vi "Balance.vi"(8 "Start Time":dbl, 10 "Boolean":bool) -> ()   [LabVIEW 2020]
uses:
  Robot Global Data.vi
  <vilib>/Rock Robotics/WPI/Utilities/WPI_GetSetVariantRefNum.vi
  <vilib>/Rock Robotics/WPI/RobotDrive/WPI_RobotDriveArcadeDrive_Standard(NoSaturation).vi
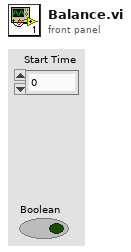
[diagram p1: front panel]
types:
  T1 = typedef "WPI_RobotDriveDevRef.ctl" = cluster{"DevStatus":errorcluster, "Motors[]":T2[], "Square Inputs":bool, "Max Output":dbl}
  T2 = typedef "WPI_MotorControlDeviceRef.ctl" = cluster{"DeviceStatus":errorcluster, "Type":T3, "PWM":cluster{"PWM Channel":T4, "DeadBand":T5}, "CAN":cluster{"Device Number":u8, "SetOutput VI Ref":variant, "GetOutput VI Ref":variant, "Enable VI Ref":variant, "Disable VI Ref":variant, "Data":variant}, "Invert":bool, "DIO PWM":cluster{"PWM \"Enable\" Channel":T4, "DIOChannel":T6, "PWM Rate":dbl}}
  T3 = typedef "WPI_MotorControlType.ctl" = enum16{"PWM", "CAN", "DIO PWM"}
  T4 = typedef "FPGA_DIOPWMChannel.ctl" = enum8{"PWM 0", "PWM 1", "PWM 2", "PWM 3", "PWM 4", "PWM 5", "PWM 6", "PWM 7", "PWM 8", "PWM 9", "PWM MXP 0", "PWM MXP 1", "PWM MXP 2", "PWM MXP 3", "PWM MXP 4", "PWM MXP 5", "PWM MXP 6", "PWM MXP 7", "PWM MXP 8", "PWM MXP 9", "Invalid"}
  T5 = typedef "WPI_PWMDeadband.ctl" = cluster{"Name":string, "maxPositivePwm":i32, "minPositivePwm":i32, "centerPwm":i32, "maxNegativePwm":i32, "minNegativePwm":i32, "angularRange":u16}
  T6 = typedef "FPGA_DIOChannel.ctl" = enum8{"DIO 0", "DIO 1", "DIO 2", "DIO 3", "DIO 4", "DIO 5", "DIO 6", "DIO 7", "DIO 8", "DIO 9", "DIO MXP 0", "DIO MXP 1", "DIO MXP 2", "DIO MXP 3", "DIO MXP 4", "DIO MXP 5", "DIO MXP 6", "DIO MXP 7", "DIO MXP 8", "DIO MXP 9", "DIO MXP 10", "DIO MXP 11", "DIO MXP 12", "DIO MXP 13", "DIO MXP 14", "DIO MXP 15", "SPI Port CS1", "SPI Port CS2", "SPI Port CS3", "SPI Port MISO", "SPI Port MOSI", "Invalid"}
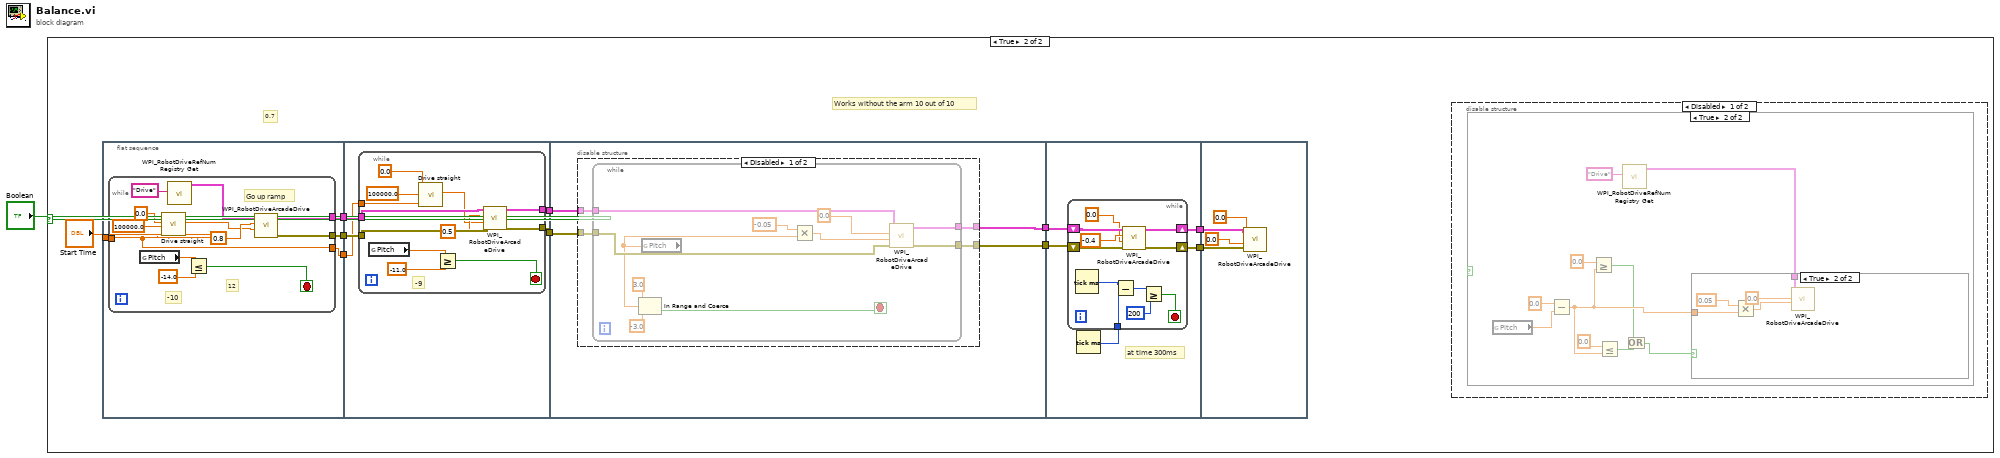
[diagram p0: block diagram]
diagram:
  n1 = case shown="True" "Boolean" {
    frame False {
    }
    frame True {
      # "0.7"
      # "Works without the arm 10 out of 10"
      n2 = flat-sequence {
        tunnel: [w30] -> w11
        tunnel: [w29] -> w10
        tunnel: "Start Time" -> [w28]
        tunnel: [w27] -> w6
        tunnel: [w47] -> w9
        tunnel: w11 -> [w46]
        tunnel: w10 -> [w45]
        tunnel: [w44] -> w8
        tunnel: w6 -> [w43]
        tunnel: w9 -> [w63]
        tunnel: w8 -> [w62]
        tunnel: [w61] -> w5
        tunnel: [w60] -> w4
        tunnel: w5 -> [w84]
        tunnel: w4 -> [w85]
        tunnel: [w83] -> w3
        tunnel: [w82] -> w2
        tunnel: w3 -> [w98]
        tunnel: w2 -> [w97]
        frame #0 {
          n3 = while {
            tunnel: [w37] -> w30
            tunnel: [w36] -> w29
            tunnel: w28 -> [w33]
            tunnel: [w33] -> w27
            stop <- w39 stop-if-true
            # "12"
            # "Go up ramp"
            # "-10"
            n4 = global read "Robot Global Data.vi" "Pitch"() -> (w40:dbl)
            n5 = call "Drive straight.vi"("Start Time"=w33, "Length(seconds)"=100000.0, "Desired angle"=0.0) -> ("X Power"=w31:dbl)  [unwired: 7 in, 1 out]
            n6 = call <vilib>:"WPI_RobotDriveRefNum Registry Get.vi"("refnum name"="Drive") -> ("RobotDriveDevRef"=w41:T1)  [unwired: 9 in, 1 out]
            n7 = Less Or Equal?(x=w40, y=-14.0) -> (x <= y?=w39:bool)
            n8 = call-poly <vilib>:"WPI_RobotDriveArcadeDrive.vi"("Y axis value"=w31, "X axis value"=0.8 ("Y axis value"), "RobotDriveDevRef"=w41) -> ("error out"=w36:errorcluster, "RobotDriveDevRef"=w37:T1)  [unwired: 6 in, 1 out]
          }
        }
        frame #1 {
          n9 = while {
            tunnel: [w57] -> w47
            tunnel: w46 -> [w56]
            tunnel: w45 -> [w55]
            tunnel: [w53] -> w44
            tunnel: w43 -> [w51]
            stop <- w59 stop-if-true
            # "-9"
            n10 = global read "Robot Global Data.vi" "Pitch"() -> (w54:dbl)
            n11 = call "Drive straight.vi"("Start Time"=w51, "Length(seconds)"=100000.0, "Desired angle"=0.0) -> ("X Power"=w48:dbl)  [unwired: 7 in, 1 out]
            n12 = Greater Or Equal?(x=w54, y=-11.0) -> (x >= y?=w59:bool)
            n13 = call-poly <vilib>:"WPI_RobotDriveArcadeDrive.vi"("error in (no error)"=w55, "Y axis value"=w48, "X axis value"=0.5 ("Y axis value"), "RobotDriveDevRef"=w56) -> ("error out"=w53:errorcluster, "RobotDriveDevRef"=w57:T1)  [unwired: 5 in, 1 out]
          }
        }
        frame #2 {
          n14 = disable-structure shown="Disabled" {
            disable-tunnel: w63 -> [w67 w80]
            disable-tunnel: w62 -> [w66 w79]
            disable-tunnel: [w65 w79] -> w61
            disable-tunnel: [w64 w80] -> w60
            frame Disabled {
              n15 = while {
                tunnel: w67 -> [w78]
                tunnel: w66 -> [w77]
                tunnel: [w76] -> w65
                tunnel: [w75] -> w64
                stop <- w74 stop-if-true
                n16 = global read "Robot Global Data.vi" "Pitch"() -> (w71:dbl)
                n17 = In Range and Coerce(upper limit=3.0, x=w71, lower limit=-3.0) -> (In Range?=w74:bool)  [unwired: 1 out]
                n18 = Multiply(x=-0.05, y=w71) -> (x*y=w70:dbl)
                n19 = call-poly <vilib>:"WPI_RobotDriveArcadeDrive.vi"("error in (no error)"=w77, "Y axis value"=w70, "X axis value"=0.0, "RobotDriveDevRef"=w78) -> ("error out"=w76:errorcluster, "RobotDriveDevRef"=w75:T1)  [unwired: 5 in, 1 out]
              }
            }
            frame Enabled {
            }
          }
        }
        frame #3 {
          # "at time 300ms"
          n20 = Tick Count (ms)() -> (millisecond timer value=w81:u32)
          n21 = while {
            shift-right: [w94] -> w83
            shift-left: w85 -> [w96]
            shift-right: [w93] -> w82
            shift-left: w84 -> [w95]
            tunnel: w81 -> [w91]
            stop <- w88 stop-if-true
            n22 = Tick Count (ms)() -> (millisecond timer value=w92:u32)
            n23 = Subtract(x=w92, y=w91) -> (x-y=w90:u32)
            n24 = call-poly <vilib>:"WPI_RobotDriveArcadeDrive.vi"("error in (no error)"=w95, "Y axis value"=0.0 ("X axis value"), "X axis value"=-0.4 ("Y axis value"), "RobotDriveDevRef"=w96) -> ("error out"=w93:errorcluster, "RobotDriveDevRef"=w94:T1)  [unwired: 5 in, 1 out]
            n25 = Greater Or Equal?(x=w90, y=u32 200) -> (x >= y?=w88:bool)
          }
        }
        frame #4 {
          n26 = call-poly <vilib>:"WPI_RobotDriveArcadeDrive.vi"("error in (no error)"=w97, "Y axis value"=0.0, "X axis value"=0.0, "RobotDriveDevRef"=w98) -> ()  [unwired: 5 in, 3 out]
        }
      }
      n27 = disable-structure shown="Disabled" {
        frame Disabled {
          n28 = case shown="True" {
            selector: _ -> [_ _]
            frame False {
            }
            frame True {
              n29 = global read "Robot Global Data.vi" "Pitch"() -> (w20:dbl)
              n30 = Subtract(x=0.0, y=w20) -> (x-y=w18:dbl)
              n31 = Greater Or Equal?(x=0.0, y=w18) -> (x >= y?=w14:bool)
              n32 = Less Or Equal?(x=0.0, y=w18) -> (x <= y?=w15:bool)
              n33 = call <vilib>:"WPI_RobotDriveRefNum Registry Get.vi"("refnum name"="Drive") -> ("RobotDriveDevRef"=w12:T1)  [unwired: 9 in, 1 out]
              n34 = Or(x=w14, y=w15) -> (x .or. y?=w16:bool)
              n35 = case shown="True" w16 {
                tunnel: w18 -> [_ w26]
                tunnel: w12 -> [_ w22]
                frame False {
                }
                frame True {
                  n36 = Multiply(x=0.05, y=w26) -> (x*y=w25:dbl)
                  n37 = call-poly <vilib>:"WPI_RobotDriveArcadeDrive.vi"("Y axis value"=w25, "X axis value"=0.0, "RobotDriveDevRef"=w22) -> ()  [unwired: 6 in, 3 out]
                }
              }
            }
          }
        }
        frame Enabled {
        }
      }
    }
  }
